vi "sensoren en motor.vi"() -> ()   [LabVIEW 2019]
uses:
  <vilib>/myRIO/Express VI/Onboard IO/AO/AO Express VI.xnode
  <vilib>/myRIO/Instrument Drivers/Onboard IO/AO/typedefs/AO Reference.ctl
  <vilib>/myRIO/Instrument Drivers/Onboard IO/AO/AO.lvlib
  <vilib>/myRIO/Common/Instrument Driver Framework/Utilities/typedefs/Analog Scaling Constants List.ctl
  <vilib>/myRIO/Common/Instrument Driver Framework/Utilities/typedefs/Analog Scaling Constants.ctl
  <vilib>/myRIO/Common/Instrument Driver Framework/myRIO v1.0/AO/typedefs/AO Channels List.ctl
  <vilib>/myRIO/Common/Instrument Driver Framework/myRIO v1.0/AO/typedefs/AO Channels Enum.ctl
  <vilib>/myRIO/Common/Instrument Driver Framework/Utilities/typedefs/myRIO Generic Hardware Reference.ctl
  <vilib>/myRIO/Common/Instrument Driver Framework/Utilities/typedefs/myRIO v1.0 Reference.ctl
  <vilib>/myRIO/Common/Instrument Driver Framework/Utilities/typedefs/Generic FPGA Reference.ctl
  <vilib>/myRIO/Common/Instrument Driver Framework/Utilities/typedefs/Hardware Version Enum.ctl
  <vilib>/myRIO/Instrument Drivers/Onboard IO/AO/vis/Write.vi
  <vilib>/myRIO/Instrument Drivers/Onboard IO/AO/vis/myRIO AO Open.xnode
  <vilib>/userDefined/High Color/nirio_resource_hc.ctl
  <vilib>/myRIO/Common/Instrument Driver Framework/myRIO v1.0/AO/vis/myRIO v1.1 Open AO.vi
  <vilib>/myRIO/Common/Instrument Driver Framework/Utilities/vis/Is FPGA Ref Available.vi
panel:
  in  "licht groen":bool
  out "Array 2":i32[](array[numeric])
  in  "input array   4":dbl[](array[numeric])
  in  "Numeric 3":dbl
  in  "Numeric 5":dbl
  in  "Numeric 4":dbl
  out "Numeric":i32
  out "x+y":i32
  in  "input array   3":dbl[](array[numeric])
  out "motor  stilleggen 2":bool
  out "motor zwak rechts sneller   2":bool
  out "motor naar links sneller 2":bool
  out "motor zeer sterk links sneller  2":bool
  out "motoren sterk rechts sneller 2":bool
  out "motor sterk links sneller   2":bool
  out "motor zwak naar links sneller  2":bool
  out "motor  zeer sterk rechts sneller 2":bool
  out "motor naar rechts sneller  2":bool
  out "Array":i32[](array[numeric])
  in  "input array   2":dbl[](array[numeric])
  out "motor naar links sneller":bool
  out "motor  zeer sterk links sneller":bool
  out "motor zwak naar rechts sneller":bool
  out "motor sterk rechts sneller":bool
  out "motoren sterk links sneller":bool
  out "motor zeer sterk rechts sneller":bool
  out "motor naar rechts sneller":bool
  out "motor zwak links sneller":bool
  out "motor  stilleggen":bool
  out "In Range? 2":bool
  out "output array":i32[](array[numeric])
  out "element":i32
  out "output array  2":i32[](array[numeric])
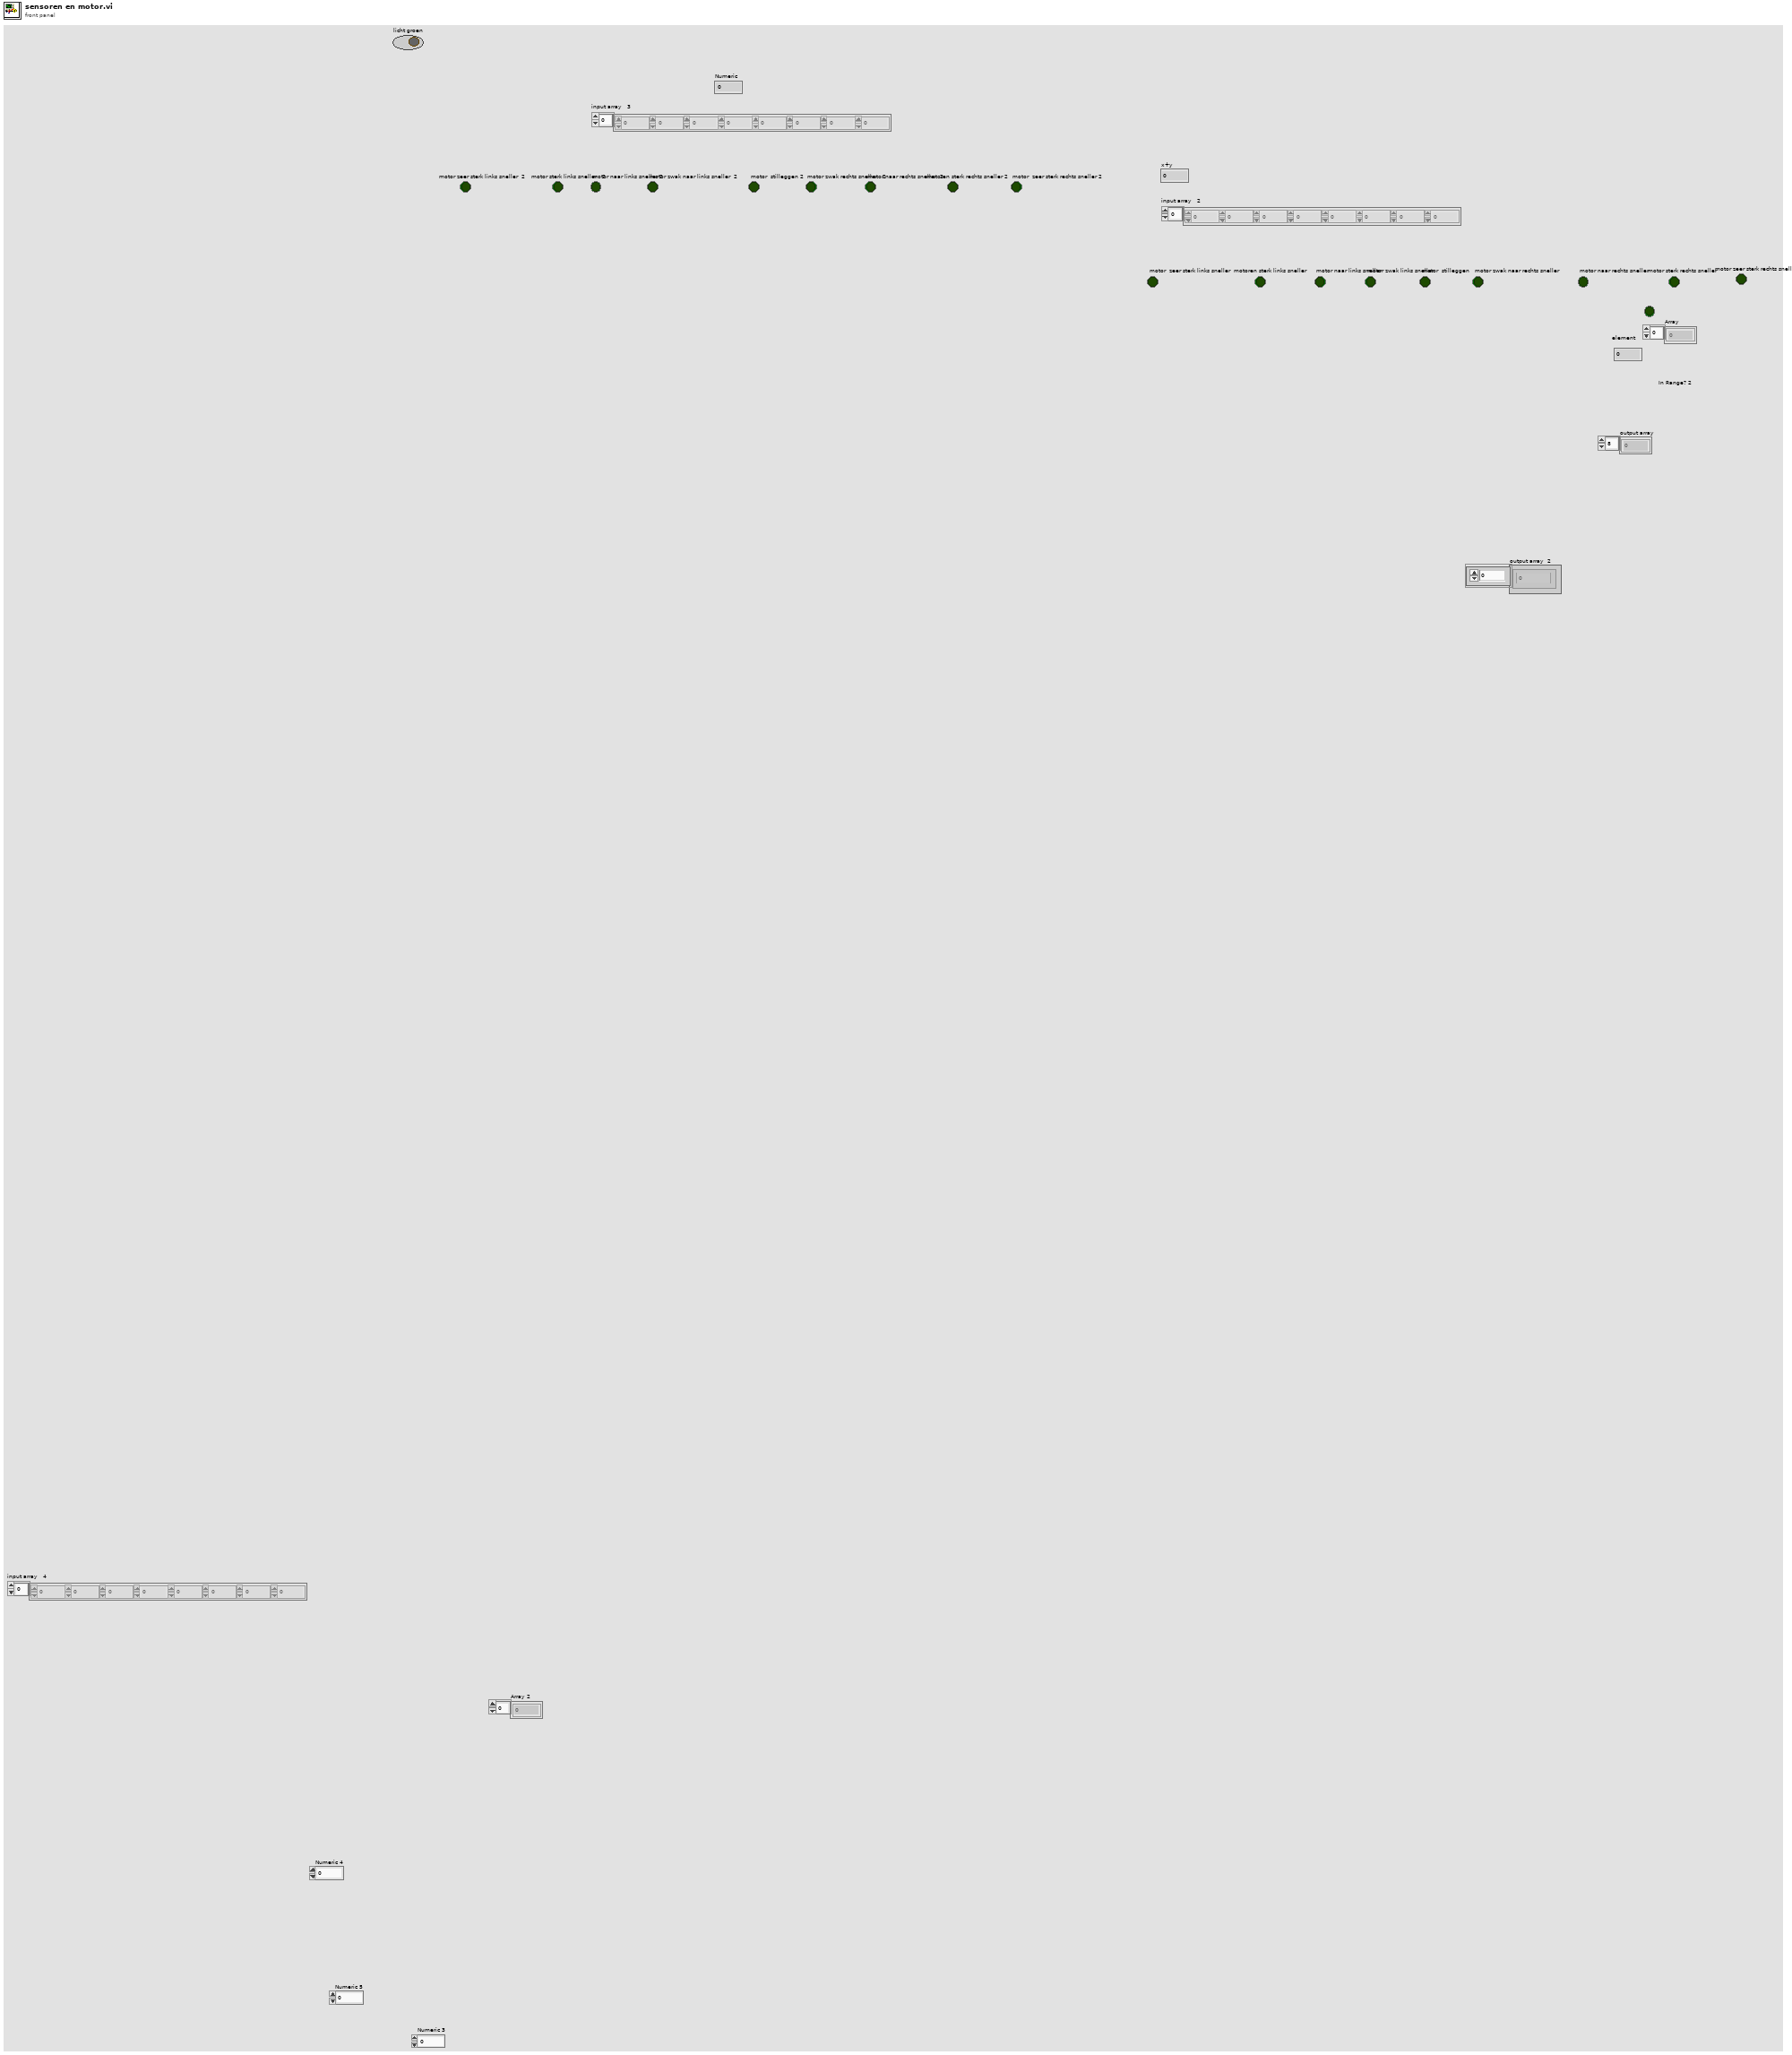
[diagram p1: front panel]
types:
  T1 = typedef "AO.lvlib/AO Reference.ctl" = cluster{"myRIO Reference":T2, "AO Channel List":T6, "AO Scaling Constant List":T8}
  T2 = typedef "myRIO Generic Hardware Reference.ctl" = cluster{"myRIO Model":T3, "myRIO Hardware Reference":T4}
  T3 = typedef "Hardware Version Enum.ctl" = enum16{"Unknown", "myRIO-1900", "myRIO-1950", "roboRIO", "NI ELVIS RIO CM", "ELVIS III"}
  T4 = typedef "myRIO v1.0 Reference.ctl" = cluster{"Generic FPGA Reference":T5, "Allow multiple opens":bool}
  T5 = typedef "Generic FPGA Reference.ctl" = refnum<k20>
  T6 = typedef "AO Channels List.ctl" = T7[]
  T7 = typedef "AO Channels Enum.ctl" = enum16{"Not Connected", "AudioOut/Left", "AudioOut/Right", "C/AO0", "C/AO1", "A/AO0", "A/AO1", "B/AO0", "B/AO1"}
  T8 = typedef "Analog Scaling Constants List.ctl" = T9[]
  T9 = typedef "Analog Scaling Constants.ctl" = cluster{"LSB Weight (Volts)":dbl, "Offset (Volts)":dbl, "Signed?":bool}
  T10 = typedef "nirio_resource_hc.ctl" = tag
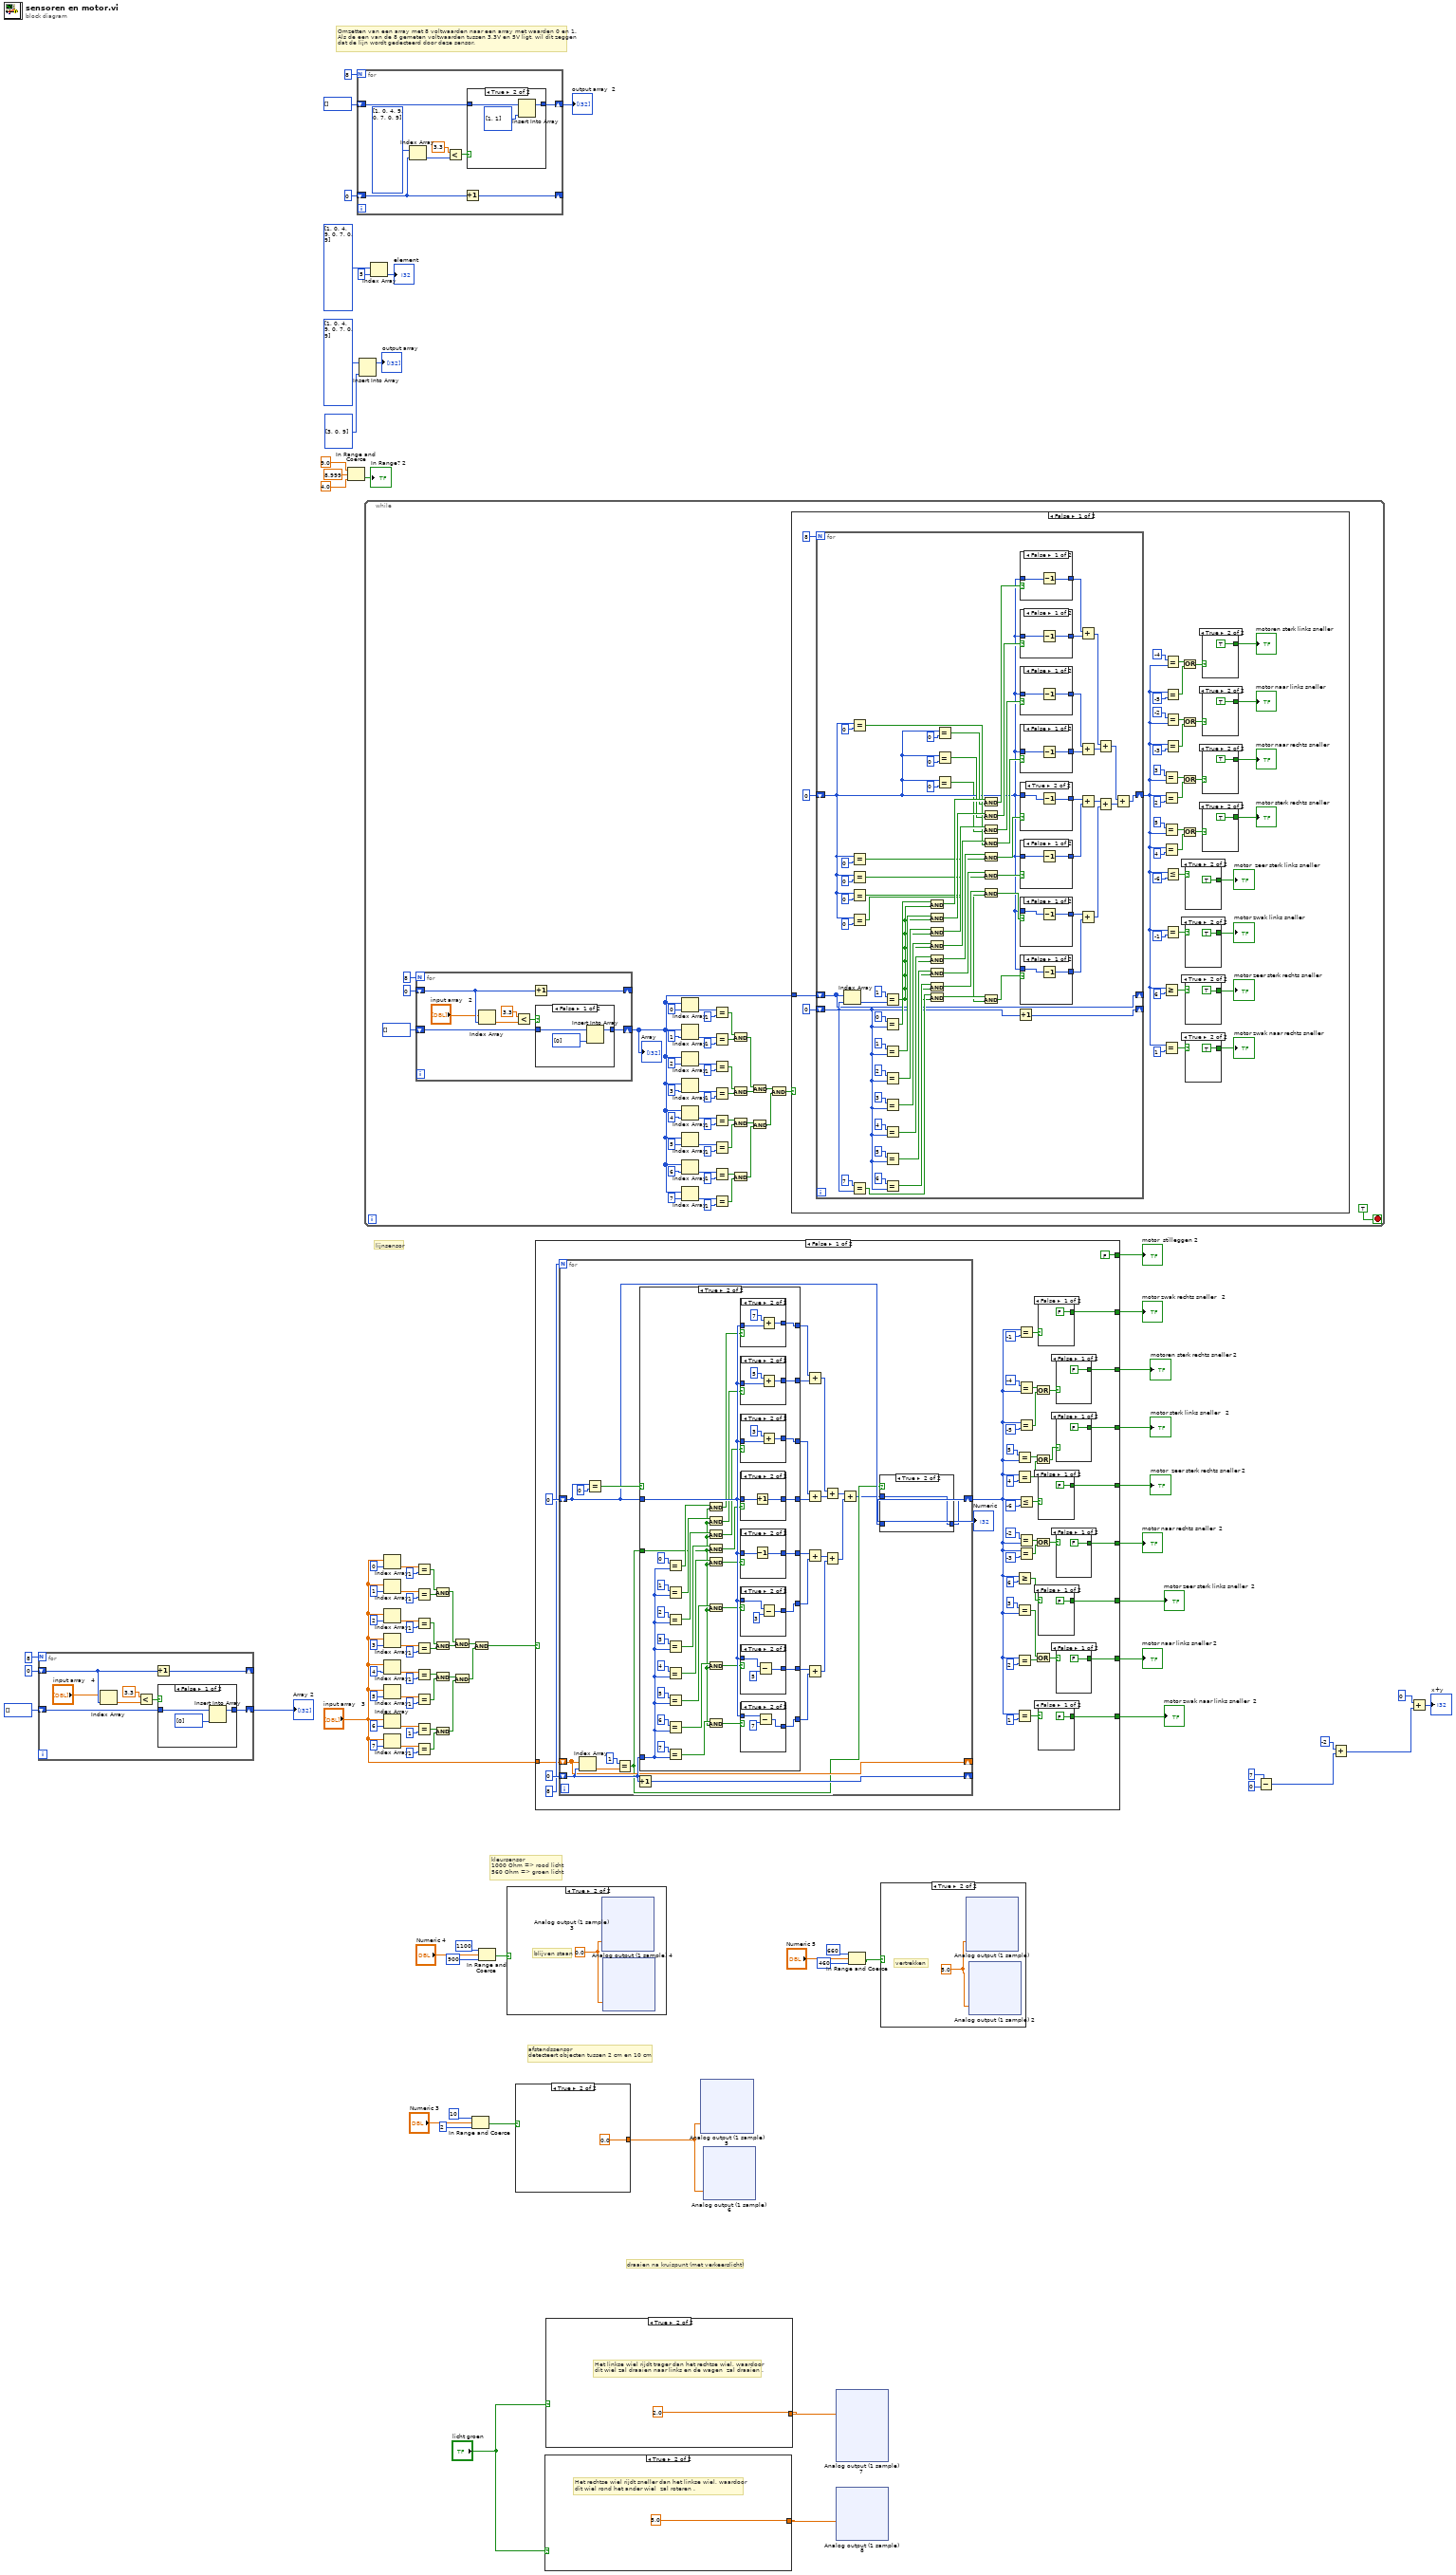
[diagram p0: block diagram]
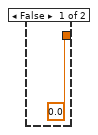
[diagram p2: hidden frame]
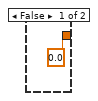
[diagram p3: hidden frame]
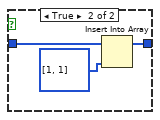
[diagram p4: hidden frame]
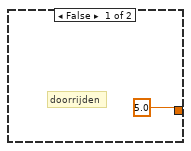
[diagram p5: hidden frame]
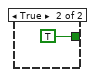
[diagram p8: hidden frame]
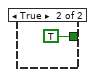
[diagram p9: hidden frame]
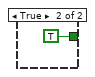
[diagram p10: hidden frame]
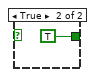
[diagram p11: hidden frame]
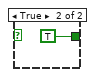
[diagram p12: hidden frame]
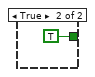
[diagram p13: hidden frame]
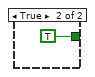
[diagram p14: hidden frame]
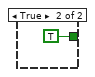
[diagram p15: hidden frame]
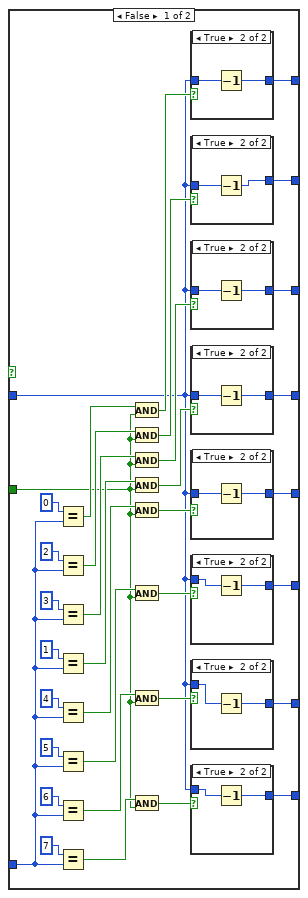
[diagram p17: hidden frame]
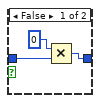
[diagram p18: hidden frame]
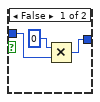
[diagram p19: hidden frame]
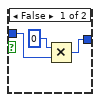
[diagram p20: hidden frame]
diagram:
  # "Omzetten van een array met 8 voltwaarden naar een array met waarden 0 en 1.\nAls de een van de 8 gemeten voltwaarden tussen 3,3V en 5V ligt, wil dit zeggen \ndat de lijn wordt gedecteerd door deze sensor."
  # "draaien na kruispunt (met verkeerslicht)"
  # "lijnsensor"
  # "kleursensor    \n1000 Ohm => rood licht\n560 Ohm => groen licht"
  # "afstandssensor\ndetecteert objecten tussen 2 cm en 10 cm"
  n1 = for {
    N: 8 -> [_]
    shift-right: [w97] -> w4
    shift-left: i32[] [] -> [w98]
    shift-right: [w94] -> _
    shift-left: 0 -> [w93]
    n2 = Index Array(array="input array   4", index=w93) -> (element=w91:dbl)
    n3 = Less?(x=3.3, y=w91) -> (x < y?=w96:bool)
    n4 = Increment(x=w93) -> (x+1=w94:i32)
    n5 = case shown="False" w96 {
      tunnel: w98 -> [w100 w102]
      tunnel: [w101 w104] -> w97
      frame False {
        n6 = Insert Into Array(array=w100, new element=i32[] [0]) -> (w101:i32[])  [unwired: 1 in]
      }
      frame True {
        n7 = Insert Into Array(array=w102, new element=i32[] [1, 1]) -> (w104:i32[])  [unwired: 1 in]
      }
    }
  }
  "Array 2" <- w4
  n8 = In Range and Coerce(upper limit=9.0, x=8.999, lower limit=4.0) -> (In Range?=→"In Range? 2":bool)  [unwired: 1 out]
  n9 = for {
    N: 8 -> [_]
    shift-right: [w111] -> w89
    shift-left: i32[] [] -> [w112]
    shift-right: [w106] -> _
    shift-left: 0 -> [w105]
    n10 = Index Array(array=i32[] [1, 0, 4, 9, 0, 7, 0, 9], index=w105) -> (element=w108:i32)
    n11 = Less?(x=3.3, y=w108) -> (x < y?=w110:bool)
    n12 = Increment(x=w105) -> (x+1=w106:i32)
    n13 = case shown="True" w110 {
      tunnel: w112 -> [w114 w116]
      tunnel: [w115 w118] -> w111
      frame False {
        n14 = Insert Into Array(array=w114, new element=i32[] [0]) -> (w115:i32[])  [unwired: 1 in]
      }
      frame True {
        n15 = Insert Into Array(array=w116, new element=i32[] [1, 1]) -> (w118:i32[])  [unwired: 1 in]
      }
    }
  }
  "output array  2" <- w89
  n16 = Insert Into Array(array=i32[] [1, 0, 4, 9, 0, 7, 0, 9], new element=i32[] [3, 0, 9]) -> (→"output array":i32[])  [unwired: 1 in]
  n17 = while {
    stop <- TRUE stop-if-true
    n18 = for {
      N: 8 -> [_]
      shift-right: [w169] -> w119
      shift-left: i32[] [] -> [w170]
      shift-right: [w166] -> _
      shift-left: 0 -> [w165]
      n19 = Index Array(array="input array   2", index=w165) -> (element=w163:dbl)
      n20 = Less?(x=3.3, y=w163) -> (x < y?=w168:bool)
      n21 = Increment(x=w165) -> (x+1=w166:i32)
      n22 = case shown="False" w168 {
        tunnel: w170 -> [w172 w174]
        tunnel: [w173 w176] -> w169
        frame False {
          n23 = Insert Into Array(array=w172, new element=i32[] [0]) -> (w173:i32[])  [unwired: 1 in]
        }
        frame True {
          n24 = Insert Into Array(array=w174, new element=i32[] [1, 1]) -> (w176:i32[])  [unwired: 1 in]
        }
      }
    }
    "Array" <- w119
    n25 = Index Array(array=w119, index=0) -> (element=w141:i32)
    n26 = Index Array(array=w119, index=1) -> (element=w162:i32)
    n27 = Index Array(array=w119, index=2) -> (element=w156:i32)
    n28 = Index Array(array=w119, index=3) -> (element=w159:i32)
    n29 = Index Array(array=w119, index=4) -> (element=w153:i32)
    n30 = Index Array(array=w119, index=5) -> (element=w150:i32)
    n31 = Index Array(array=w119, index=6) -> (element=w147:i32)
    n32 = Index Array(array=w119, index=7) -> (element=w144:i32)
    n33 = Equal?(x=w141, y=1) -> (x = y?=w138:bool)
    n34 = Equal?(x=w162, y=1) -> (x = y?=w137:bool)
    n35 = Equal?(x=w156, y=1) -> (x = y?=w136:bool)
    n36 = Equal?(x=w159, y=1) -> (x = y?=w135:bool)
    n37 = Equal?(x=w153, y=1) -> (x = y?=w134:bool)
    n38 = Equal?(x=w150, y=1) -> (x = y?=w133:bool)
    n39 = Equal?(x=w147, y=1) -> (x = y?=w132:bool)
    n40 = Equal?(x=w144, y=1) -> (x = y?=w131:bool)
    n41 = And(x=w138, y=w137) -> (x .and. y?=w130:bool)
    n42 = And(x=w136, y=w135) -> (x .and. y?=w129:bool)
    n43 = And(x=w134, y=w133) -> (x .and. y?=w128:bool)
    n44 = And(x=w132, y=w131) -> (x .and. y?=w127:bool)
    n45 = And(x=w130, y=w129) -> (x .and. y?=w126:bool)
    n46 = And(x=w128, y=w127) -> (x .and. y?=w125:bool)
    n47 = And(x=w126, y=w125) -> (x .and. y?=w124:bool)
    n48 = case shown="False" w124 {
      tunnel: w119 -> [w177 _]
      frame False {
        n49 = for {
          N: 8 -> [_]
          shift-right: [w303] -> _
          shift-left: 0 -> [w284]
          shift-right: [w269] -> w179
          shift-left: 0 -> [w237]
          shift-right: [w234] -> _
          shift-left: w177 -> [w234]
          n50 = Index Array(array=w234, index=w284) -> (element=w235:i32)
          n51 = Equal?(x=w237, y=0) -> (x = y?=w243:bool)
          n52 = Equal?(x=w237, y=0) -> (x = y?=w247:bool)
          n53 = Equal?(x=w237, y=0) -> (x = y?=w249:bool)
          n54 = Equal?(x=w237, y=0) -> (x = y?=w245:bool)
          n55 = Equal?(x=w237, y=0) -> (x = y?=w251:bool)
          n56 = Equal?(x=7, y=w284) -> (x = y?=w296:bool)
          n57 = Equal?(x=1, y=w235) -> (x = y?=w285:bool)
          n58 = Equal?(x=0, y=w284) -> (x = y?=w294:bool)
          n59 = Equal?(x=1, y=w284) -> (x = y?=w286:bool)
          n60 = Equal?(x=2, y=w284) -> (x = y?=w300:bool)
          n61 = Equal?(x=3, y=w284) -> (x = y?=w301:bool)
          n62 = Equal?(x=4, y=w284) -> (x = y?=w298:bool)
          n63 = Equal?(x=5, y=w284) -> (x = y?=w299:bool)
          n64 = Equal?(x=6, y=w284) -> (x = y?=w297:bool)
          n65 = And(x=w294, y=w285) -> (x .and. y?=w268:bool)
          n66 = And(x=w286, y=w285) -> (x .and. y?=w265:bool)
          n67 = And(x=w300, y=w285) -> (x .and. y?=w263:bool)
          n68 = And(x=w301, y=w285) -> (x .and. y?=w261:bool)
          n69 = And(x=w298, y=w285) -> (x .and. y?=w260:bool)
          n70 = And(x=w299, y=w285) -> (x .and. y?=w258:bool)
          n71 = And(x=w297, y=w285) -> (x .and. y?=w256:bool)
          n72 = And(x=w296, y=w285) -> (x .and. y?=w253:bool)
          n73 = Equal?(x=w237, y=0) -> (x = y?=w241:bool)
          n74 = Equal?(x=w237, y=0) -> (x = y?=w239:bool)
          n75 = Equal?(x=w237, y=0) -> (x = y?=w236:bool)
          n76 = And(x=w268, y=w241) -> (x .and. y?=w267:bool)
          n77 = And(x=w265, y=w239) -> (x .and. y?=w266:bool)
          n78 = And(x=w263, y=w236) -> (x .and. y?=w264:bool)
          n79 = And(x=w261, y=w243) -> (x .and. y?=w262:bool)
          n80 = And(x=w260, y=w247) -> (x .and. y?=w259:bool)
          n81 = And(x=w258, y=w249) -> (x .and. y?=w257:bool)
          n82 = And(x=w256, y=w245) -> (x .and. y?=w255:bool)
          n83 = And(x=w253, y=w251) -> (x .and. y?=w254:bool)
          n84 = Increment(x=w284) -> (x+1=w303:i32)
          n85 = case shown="False" w267 {
            tunnel: w237 -> [w304 w307]
            tunnel: [w305 w306] -> w283
            frame False {
              n86 = Decrement(x=w304) -> (x-1=w305:i32)
            }
            frame True {
              n87 = Add(x=7, y=w307) -> (x+y=w306:i32)
            }
          }
          n88 = case shown="False" w266 {
            tunnel: w237 -> [w337 w339]
            tunnel: [w338 w340] -> w282
            frame False {
              n89 = Decrement(x=w337) -> (x-1=w338:i32)
            }
            frame True {
              n90 = Add(x=5, y=w339) -> (x+y=w340:i32)
            }
          }
          n91 = case shown="False" w264 {
            tunnel: w237 -> [w332 w335]
            tunnel: [w333 w334] -> w281
            frame False {
              n92 = Decrement(x=w332) -> (x-1=w333:i32)
            }
            frame True {
              n93 = Add(x=3, y=w335) -> (x+y=w334:i32)
            }
          }
          n94 = case shown="False" w262 {
            tunnel: w237 -> [w328 w331]
            tunnel: [w329 w330] -> w280
            frame False {
              n95 = Decrement(x=w328) -> (x-1=w329:i32)
            }
            frame True {
              n96 = Increment(x=w331) -> (x+1=w330:i32)
            }
          }
          n97 = case shown="True" w259 {
            tunnel: w237 -> [w324 w327]
            tunnel: [w325 w326] -> w279
            frame False {
              n98 = Increment(x=w324) -> (x+1=w325:i32)
            }
            frame True {
              n99 = Decrement(x=w327) -> (x-1=w326:i32)
            }
          }
          n100 = case shown="False" w257 {
            tunnel: w237 -> [w314 w316]
            tunnel: [w315 w317] -> w278
            frame False {
              n101 = Decrement(x=w314) -> (x-1=w315:i32)
            }
            frame True {
              n102 = Subtract(x=3, y=w316) -> (x-y=w317:i32)
            }
          }
          n103 = case shown="False" w255 {
            tunnel: w237 -> [w319 w322]
            tunnel: [w320 w321] -> w277
            frame False {
              n104 = Decrement(x=w319) -> (x-1=w320:i32)
            }
            frame True {
              n105 = Subtract(x=5, y=w322) -> (x-y=w321:i32)
            }
          }
          n106 = case shown="False" w254 {
            tunnel: w237 -> [w310 w312]
            tunnel: [w309 w311] -> w276
            frame False {
              n107 = Decrement(x=w310) -> (x-1=w309:i32)
            }
            frame True {
              n108 = Subtract(x=7, y=w312) -> (x-y=w311:i32)
            }
          }
          n109 = Add(x=w283, y=w282) -> (x+y=w273:i32)
          n110 = Add(x=w281, y=w280) -> (x+y=w272:i32)
          n111 = Add(x=w279, y=w278) -> (x+y=w274:i32)
          n112 = Add(x=w277, y=w276) -> (x+y=w275:i32)
          n113 = Add(x=w273, y=w272) -> (x+y=w271:i32)
          n114 = Add(x=w274, y=w275) -> (x+y=w270:i32)
          n115 = Add(x=w271, y=w270) -> (x+y=w269:i32)
        }
        n116 = Equal?(x=3, y=w179) -> (x = y?=w195:bool)
        n117 = Equal?(x=w179, y=2) -> (x = y?=w196:bool)
        n118 = Equal?(x=5, y=w179) -> (x = y?=w199:bool)
        n119 = Equal?(x=w179, y=4) -> (x = y?=w200:bool)
        n120 = Greater Or Equal?(x=w179, y=6) -> (x >= y?=w204:bool)
        n121 = Equal?(x=w179, y=1) -> (x = y?=w213:bool)
        n122 = Equal?(x=-4, y=w179) -> (x = y?=w185:bool)
        n123 = Equal?(x=w179, y=-5) -> (x = y?=w186:bool)
        n124 = Equal?(x=-2, y=w179) -> (x = y?=w189:bool)
        n125 = Equal?(x=w179, y=-3) -> (x = y?=w190:bool)
        n126 = Less Or Equal?(x=w179, y=-6) -> (x <= y?=w181:bool)
        n127 = Equal?(x=w179, y=-1) -> (x = y?=w183:bool)
        n128 = Or(x=w185, y=w186) -> (x .or. y?=w178:bool)
        n129 = Or(x=w189, y=w190) -> (x .or. y?=w182:bool)
        n130 = Or(x=w195, y=w196) -> (x .or. y?=w193:bool)
        n131 = Or(x=w199, y=w200) -> (x .or. y?=w201:bool)
        n132 = case shown="True" w181 {
          tunnel: [FALSE ("Boolean 2") TRUE ("Boolean 2")] -> w206
          frame False {
          }
          frame True {
          }
        }
        "motor  zeer sterk links sneller" <- w206
        n133 = case shown="True" w183 {
          tunnel: [FALSE ("Boolean 2") TRUE ("Boolean 2")] -> w208
          frame False {
          }
          frame True {
          }
        }
        "motor zwak links sneller" <- w208
        n134 = case shown="True" w204 {
          tunnel: [FALSE ("Boolean 2") TRUE ("Boolean 2")] -> w212
          frame False {
          }
          frame True {
          }
        }
        "motor zeer sterk rechts sneller" <- w212
        n135 = case shown="True" w213 {
          tunnel: [FALSE ("Boolean 2") TRUE ("Boolean 2")] -> w209
          frame False {
          }
          frame True {
          }
        }
        "motor zwak naar rechts sneller" <- w209
        n136 = case shown="True" w178 {
          tunnel: [FALSE ("Boolean 2") TRUE ("Boolean 2")] -> w207
          frame False {
          }
          frame True {
          }
        }
        "motoren sterk links sneller" <- w207
        n137 = case shown="True" w182 {
          tunnel: [FALSE ("Boolean 2") TRUE ("Boolean 2")] -> w205
          frame False {
          }
          frame True {
          }
        }
        "motor naar links sneller" <- w205
        n138 = case shown="True" w193 {
          tunnel: [FALSE ("Boolean 2") TRUE ("Boolean 2")] -> w210
          frame False {
          }
          frame True {
          }
        }
        "motor naar rechts sneller" <- w210
        n139 = case shown="True" w201 {
          tunnel: [FALSE ("Boolean 2") TRUE ("Boolean 2")] -> w211
          frame False {
          }
          frame True {
          }
        }
        "motor sterk rechts sneller" <- w211
      }
      frame True {
        "motor  stilleggen" <- TRUE ("Boolean 2")
      }
    }
  }
  n140 = Index Array(array=i32[] [1, 0, 4, 9, 0, 7, 0, 9], index=5) -> (element=→"element":i32)
  n141 = Index Array(array="input array   3", index=0) -> (element=w55:dbl)
  n142 = Index Array(array="input array   3", index=1) -> (element=w76:dbl)
  n143 = Index Array(array="input array   3", index=2) -> (element=w70:dbl)
  n144 = Index Array(array="input array   3", index=3) -> (element=w73:dbl)
  n145 = Index Array(array="input array   3", index=4) -> (element=w67:dbl)
  n146 = Index Array(array="input array   3", index=5) -> (element=w64:dbl)
  n147 = Index Array(array="input array   3", index=6) -> (element=w61:dbl)
  n148 = Index Array(array="input array   3", index=7) -> (element=w58:dbl)
  n149 = Equal?(x=w55, y=1) -> (x = y?=w52:bool)
  n150 = Equal?(x=w76, y=1) -> (x = y?=w51:bool)
  n151 = Equal?(x=w70, y=1) -> (x = y?=w50:bool)
  n152 = Equal?(x=w73, y=1) -> (x = y?=w49:bool)
  n153 = Equal?(x=w67, y=1) -> (x = y?=w48:bool)
  n154 = Equal?(x=w64, y=1) -> (x = y?=w47:bool)
  n155 = Equal?(x=w61, y=1) -> (x = y?=w46:bool)
  n156 = Equal?(x=w58, y=1) -> (x = y?=w45:bool)
  n157 = And(x=w52, y=w51) -> (x .and. y?=w44:bool)
  n158 = And(x=w50, y=w49) -> (x .and. y?=w43:bool)
  n159 = And(x=w48, y=w47) -> (x .and. y?=w42:bool)
  n160 = And(x=w46, y=w45) -> (x .and. y?=w41:bool)
  n161 = And(x=w44, y=w43) -> (x .and. y?=w40:bool)
  n162 = And(x=w42, y=w41) -> (x .and. y?=w39:bool)
  n163 = In Range and Coerce(upper limit=10, x="Numeric 3", lower limit=2) -> (In Range?=w9:bool)  [unwired: 1 out]
  n164 = And(x=w40, y=w39) -> (x .and. y?=w38:bool)
  n165 = In Range and Coerce(upper limit=1100, x="Numeric 4", lower limit=900) -> (In Range?=w17:bool)  [unwired: 1 out]
  n166 = case shown="True" w17 {
    frame False {
    }
    frame True {
      w343 = 0.0
      # "blijven staan"
      n167 = xnode "Analog output (1 sample) 3"("A/AO0 (Pin 2)"=w343) -> ()  [unwired: 1 in, 1 out]
      n168 = xnode "Analog output (1 sample) 4"("A/AO0 (Pin 2)"=w343) -> ()  [unwired: 1 in, 1 out]
    }
  }
  n169 = case shown="True" w9 {
    tunnel: [5.0 0.0] -> w12
    frame False {
      # "doorrijden"
    }
    frame True {
    }
  }
  n170 = case shown="False" w38 {
    tunnel: "input array   3" -> [w430 _]
    tunnel: [FALSE ("Boolean 2") TRUE ("Boolean 2")] -> w36
    tunnel: [w428 FALSE ("Boolean 2")] -> w35
    tunnel: [w427 FALSE ("Boolean 2")] -> w34
    tunnel: [w426 FALSE ("Boolean 2")] -> w33
    tunnel: [w425 FALSE ("Boolean 2")] -> w32
    tunnel: [w424 FALSE ("Boolean 2")] -> w31
    tunnel: [w423 FALSE ("Boolean 2")] -> w30
    tunnel: [w422 FALSE ("Boolean 2")] -> w29
    tunnel: [w421 FALSE ("Boolean 2")] -> w28
    frame False {
      n171 = for {
        N: 8 -> [_]
        shift-right: [w488] -> _
        shift-left: 0 -> [w502]
        shift-right: [w480] -> w420
        shift-left: 0 -> [w481]
        shift-right: [w493] -> _
        shift-left: w430 -> [w493]
        n172 = Index Array(array=w493, index=w502) -> (element=w492:dbl)
        n173 = Equal?(x=w481, y=0) -> (x = y?=w489:bool)
        n174 = Equal?(x=1, y=w492) -> (x = y?=w479:bool)
        n175 = Increment(x=w502) -> (x+1=w488:i32)
        n176 = case shown="True" w489 {
          tunnel: w502 -> [w512 w598]
          tunnel: [w506 w597] -> w501
          tunnel: [w513 w596] -> w500
          tunnel: [w514 w595] -> w499
          tunnel: [w515 w594] -> w498
          tunnel: w481 -> [w505 w593]
          tunnel: w479 -> [w511 w584]
          tunnel: [w509 w583] -> w487
          tunnel: [w510 w582] -> w486
          tunnel: [w507 w581] -> w484
          tunnel: [w508 w580] -> w483
          frame False {
            n177 = Equal?(x=0, y=w512) -> (x = y?=w532:bool)
            n178 = Equal?(x=2, y=w512) -> (x = y?=w538:bool)
            n179 = Equal?(x=3, y=w512) -> (x = y?=w539:bool)
            n180 = Equal?(x=1, y=w512) -> (x = y?=w524:bool)
            n181 = Equal?(x=4, y=w512) -> (x = y?=w536:bool)
            n182 = Equal?(x=5, y=w512) -> (x = y?=w537:bool)
            n183 = Equal?(x=6, y=w512) -> (x = y?=w535:bool)
            n184 = Equal?(x=7, y=w512) -> (x = y?=w534:bool)
            n185 = And(x=w532, y=w511) -> (x .and. y?=w516:bool)
            n186 = And(x=w538, y=w511) -> (x .and. y?=w518:bool)
            n187 = And(x=w539, y=w511) -> (x .and. y?=w519:bool)
            n188 = And(x=w524, y=w511) -> (x .and. y?=w517:bool)
            n189 = And(x=w536, y=w511) -> (x .and. y?=w520:bool)
            n190 = And(x=w537, y=w511) -> (x .and. y?=w521:bool)
            n191 = And(x=w535, y=w511) -> (x .and. y?=w522:bool)
            n192 = And(x=w534, y=w511) -> (x .and. y?=w523:bool)
            n193 = case shown="True" w516 {
              tunnel: [w541 w544] -> w510
              tunnel: w505 -> [w540 w543]
              frame False {
                n194 = Multiply(x=0, y=w540) -> (x*y=w541:i32)
              }
              frame True {
                n195 = Decrement(x=w543) -> (x-1=w544:i32)
              }
            }
            n196 = case shown="True" w518 {
              tunnel: [w572 w573] -> w509
              tunnel: w505 -> [w571 w574]
              frame False {
                n197 = Multiply(x=0, y=w571) -> (x*y=w572:i32)
              }
              frame True {
                n198 = Decrement(x=w574) -> (x-1=w573:i32)
              }
            }
            n199 = case shown="True" w519 {
              tunnel: [w566 w569] -> w508
              tunnel: w505 -> [w565 w568]
              frame False {
                n200 = Multiply(x=0, y=w565) -> (x*y=w566:i32)
              }
              frame True {
                n201 = Decrement(x=w568) -> (x-1=w569:i32)
              }
            }
            n202 = case shown="True" w517 {
              tunnel: [w576 w579] -> w507
              tunnel: w505 -> [w575 w578]
              frame False {
                n203 = Multiply(x=0, y=w575) -> (x*y=w576:i32)
              }
              frame True {
                n204 = Decrement(x=w578) -> (x-1=w579:i32)
              }
            }
            n205 = case shown="True" w520 {
              tunnel: [w561 w564] -> w506
              tunnel: w505 -> [w560 w563]
              frame False {
                n206 = Multiply(x=0, y=w560) -> (x*y=w561:i32)
              }
              frame True {
                n207 = Decrement(x=w563) -> (x-1=w564:i32)
              }
            }
            n208 = case shown="True" w521 {
              tunnel: [w551 w554] -> w513
              tunnel: w505 -> [w550 w553]
              frame False {
                n209 = Multiply(x=0, y=w550) -> (x*y=w551:i32)
              }
              frame True {
                n210 = Decrement(x=w553) -> (x-1=w554:i32)
              }
            }
            n211 = case shown="True" w522 {
              tunnel: [w556 w559] -> w514
              tunnel: w505 -> [w555 w558]
              frame False {
                n212 = Multiply(x=0, y=w555) -> (x*y=w556:i32)
              }
              frame True {
                n213 = Decrement(x=w558) -> (x-1=w559:i32)
              }
            }
            n214 = case shown="True" w523 {
              tunnel: [w545 w549] -> w515
              tunnel: w505 -> [w546 w548]
              frame False {
                n215 = Multiply(x=0, y=w546) -> (x*y=w545:i32)
              }
              frame True {
                n216 = Decrement(x=w548) -> (x-1=w549:i32)
              }
            }
          }
          frame True {
            n217 = Equal?(x=0, y=w598) -> (x = y?=w607:bool)
            n218 = Equal?(x=1, y=w598) -> (x = y?=w599:bool)
            n219 = Equal?(x=2, y=w598) -> (x = y?=w613:bool)
            n220 = Equal?(x=3, y=w598) -> (x = y?=w614:bool)
            n221 = Equal?(x=4, y=w598) -> (x = y?=w611:bool)
            n222 = Equal?(x=5, y=w598) -> (x = y?=w612:bool)
            n223 = Equal?(x=6, y=w598) -> (x = y?=w610:bool)
            n224 = Equal?(x=7, y=w598) -> (x = y?=w609:bool)
            n225 = And(x=w607, y=w584) -> (x .and. y?=w585:bool)
            n226 = And(x=w599, y=w584) -> (x .and. y?=w586:bool)
            n227 = And(x=w613, y=w584) -> (x .and. y?=w587:bool)
            n228 = And(x=w614, y=w584) -> (x .and. y?=w588:bool)
            n229 = And(x=w611, y=w584) -> (x .and. y?=w589:bool)
            n230 = And(x=w612, y=w584) -> (x .and. y?=w590:bool)
            n231 = And(x=w610, y=w584) -> (x .and. y?=w591:bool)
            n232 = And(x=w609, y=w584) -> (x .and. y?=w592:bool)
            n233 = case shown="True" w585 {
              tunnel: w593 -> [w615 w619]
              tunnel: [w616 w618] -> w582
              frame False {
                n234 = Multiply(x=0, y=w615) -> (x*y=w616:i32)
              }
              frame True {
                n235 = Add(x=7, y=w619) -> (x+y=w618:i32)
              }
            }
            n236 = case shown="True" w586 {
              tunnel: w593 -> [w655 w658]
              tunnel: [w656 w659] -> w583
              frame False {
                n237 = Multiply(x=0, y=w655) -> (x*y=w656:i32)
              }
              frame True {
                n238 = Add(x=5, y=w658) -> (x+y=w659:i32)
              }
            }
            n239 = case shown="True" w587 {
              tunnel: w593 -> [w649 w653]
              tunnel: [w650 w652] -> w580
              frame False {
                n240 = Multiply(x=0, y=w649) -> (x*y=w650:i32)
              }
              frame True {
                n241 = Add(x=3, y=w653) -> (x+y=w652:i32)
              }
            }
            n242 = case shown="True" w588 {
              tunnel: w593 -> [w645 w648]
              tunnel: [w644 w647] -> w581
              frame False {
                n243 = Multiply(x=0, y=w645) -> (x*y=w644:i32)
              }
              frame True {
                n244 = Increment(x=w648) -> (x+1=w647:i32)
              }
            }
            n245 = case shown="True" w589 {
              tunnel: w593 -> [w639 w643]
              tunnel: [w640 w642] -> w597
              frame False {
                n246 = Multiply(x=0, y=w639) -> (x*y=w640:i32)
              }
              frame True {
                n247 = Decrement(x=w643) -> (x-1=w642:i32)
              }
            }
            n248 = case shown="True" w590 {
              tunnel: w593 -> [w628 w630]
              tunnel: [w627 w632] -> w596
              frame False {
                n249 = Multiply(x=0, y=w628) -> (x*y=w627:i32)
              }
              frame True {
                n250 = Subtract(x=w630, y=3) -> (x-y=w632:i32)
              }
            }
            n251 = case shown="True" w591 {
              tunnel: w593 -> [w634 w636]
              tunnel: [w633 w637] -> w595
              frame False {
                n252 = Multiply(x=0, y=w634) -> (x*y=w633:i32)
              }
              frame True {
                n253 = Subtract(x=w636, y=5) -> (x-y=w637:i32)
              }
            }
            n254 = case shown="True" w592 {
              tunnel: w593 -> [w621 w624]
              tunnel: [w622 w625] -> w594
              frame False {
                n255 = Multiply(x=0, y=w621) -> (x*y=w622:i32)
              }
              frame True {
                n256 = Subtract(x=w624, y=7) -> (x-y=w625:i32)
              }
            }
          }
        }
        n257 = Add(x=w486, y=w487) -> (x+y=w485:i32)
        n258 = Add(x=w483, y=w484) -> (x+y=w482:i32)
        n259 = Add(x=w501, y=w500) -> (x+y=w496:i32)
        n260 = Add(x=w499, y=w498) -> (x+y=w497:i32)
        n261 = Add(x=w485, y=w482) -> (x+y=w495:i32)
        n262 = Add(x=w496, y=w497) -> (x+y=w494:i32)
        n263 = Add(x=w495, y=w494) -> (x+y=w478:i32)
        n264 = case shown="True" w479 {
          tunnel: w481 -> [w503 _]
          tunnel: [w503 w504] -> w480
          tunnel: w478 -> [_ w504]
          frame False {
          }
          frame True {
          }
        }
      }
      "Numeric" <- w420
      n265 = Equal?(x=5, y=w420) -> (x = y?=w451:bool)
      n266 = Equal?(x=w420, y=4) -> (x = y?=w452:bool)
      n267 = Greater Or Equal?(x=w420, y=6) -> (x >= y?=w456:bool)
      n268 = Equal?(x=3, y=w420) -> (x = y?=w447:bool)
      n269 = Equal?(x=w420, y=2) -> (x = y?=w448:bool)
      n270 = Equal?(x=w420, y=1) -> (x = y?=w457:bool)
      n271 = Equal?(x=w420, y=-1) -> (x = y?=w435:bool)
      n272 = Equal?(x=-4, y=w420) -> (x = y?=w437:bool)
      n273 = Equal?(x=w420, y=-5) -> (x = y?=w438:bool)
      n274 = Less Or Equal?(x=w420, y=-6) -> (x <= y?=w433:bool)
      n275 = Equal?(x=-2, y=w420) -> (x = y?=w441:bool)
      n276 = Equal?(x=w420, y=-3) -> (x = y?=w442:bool)
      n277 = Or(x=w437, y=w438) -> (x .or. y?=w431:bool)
      n278 = Or(x=w451, y=w452) -> (x .or. y?=w453:bool)
      n279 = Or(x=w441, y=w442) -> (x .or. y?=w434:bool)
      n280 = Or(x=w447, y=w448) -> (x .or. y?=w445:bool)
      n281 = case shown="False" w435 {
        tunnel: [FALSE ("Boolean 2") TRUE ("Boolean 2")] -> w421
        frame False {
        }
        frame True {
        }
      }
      n282 = case shown="False" w433 {
        tunnel: [FALSE ("Boolean 2") TRUE ("Boolean 2")] -> w424
        frame False {
        }
        frame True {
        }
      }
      n283 = case shown="False" w456 {
        tunnel: [FALSE ("Boolean 2") TRUE ("Boolean 2")] -> w422
        frame False {
        }
        frame True {
        }
      }
      n284 = case shown="False" w457 {
        tunnel: [FALSE ("Boolean 2") TRUE ("Boolean 2")] -> w423
        frame False {
        }
        frame True {
        }
      }
      n285 = case shown="False" w431 {
        tunnel: [FALSE ("Boolean 2") TRUE ("Boolean 2")] -> w426
        frame False {
        }
        frame True {
        }
      }
      n286 = case shown="False" w453 {
        tunnel: [FALSE ("Boolean 2") TRUE ("Boolean 2")] -> w427
        frame False {
        }
        frame True {
        }
      }
      n287 = case shown="False" w434 {
        tunnel: [FALSE ("Boolean 2") TRUE ("Boolean 2")] -> w428
        frame False {
        }
        frame True {
        }
      }
      n288 = case shown="False" w445 {
        tunnel: [FALSE ("Boolean 2") TRUE ("Boolean 2")] -> w425
        frame False {
        }
        frame True {
        }
      }
    }
    frame True {
    }
  }
  "motor  stilleggen 2" <- w36
  "motor naar links sneller 2" <- w32
  "motoren sterk rechts sneller 2" <- w33
  "motor sterk links sneller   2" <- w34
  "motor naar rechts sneller  2" <- w35
  "motor zwak rechts sneller   2" <- w28
  "motor zeer sterk links sneller  2" <- w29
  "motor zwak naar links sneller  2" <- w30
  "motor  zeer sterk rechts sneller 2" <- w31
  n289 = case shown="True" "licht groen" {
    tunnel: [0.0 5.0] -> w2
    frame False {
    }
    frame True {
      # "Het rechtse wiel rijdt sneller dan het linkse wiel, waardoor \ndit wiel rond het ander wiel  zal roteren ."
    }
  }
  n290 = case shown="True" "licht groen" {
    tunnel: [0.0 2.0] -> w3
    frame False {
    }
    frame True {
      # "Het linkse wiel rijdt trager dan het rechtse wiel, waardoor \ndit wiel zal draaien naar links en de wagen  zal draaien ."
    }
  }
  n291 = xnode "Analog output (1 sample) 5"("A/AO0 (Pin 2)"=w12) -> ()  [unwired: 1 in, 1 out]
  n292 = xnode "Analog output (1 sample) 6"("A/AO0 (Pin 2)"=w12) -> ()  [unwired: 1 in, 1 out]
  n293 = xnode "Analog output (1 sample) 7"("A/AO0 (Pin 2)"=w3) -> ()  [unwired: 1 in, 1 out]
  n294 = xnode "Analog output (1 sample) 8"("A/AO0 (Pin 2)"=w2) -> ()  [unwired: 1 in, 1 out]
  n295 = In Range and Coerce(upper limit=660, x="Numeric 5", lower limit=460) -> (In Range?=w13:bool)  [unwired: 1 out]
  n296 = case shown="True" w13 {
    frame False {
    }
    frame True {
      w674 = 5.0
      # "vertrekken"
      n297 = xnode "Analog output (1 sample)"("A/AO0 (Pin 2)"=w674) -> ()  [unwired: 1 in, 1 out]
      n298 = xnode "Analog output (1 sample) 2"("A/AO0 (Pin 2)"=w674) -> ()  [unwired: 1 in, 1 out]
    }
  }
  n299 = Subtract(x=7, y=0) -> (x-y=w23:i32)
  n300 = Add(x=-2, y=w23) -> (x+y=w24:i32)
  n301 = Add(x=0, y=w24) -> (x+y=→"x+y":i32)
